vi "Initialize Multicolumn Listbox.vi"(8 "error in":errorcluster, 11 "MulticolumnListbox":refnum<vi>) -> (0 "error out":errorcluster)   [LabVIEW 2018, in "NI_TDMS File Viewer.lvlib"]
uses:
  NI_TDMS File Viewer.lvlib
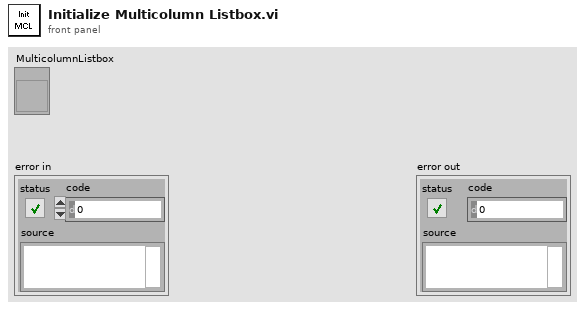
[diagram p1: front panel]
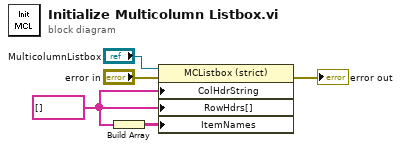
[diagram p0: block diagram]
diagram:
  w3 = string[] [] ("Column Header Strings[]")
  n1 = Build Array(w3) -> (w2:string[][])
  n2 = property on="Property Node" class="MCListbox (strict)"(reference="MulticolumnListbox", error in="error in", "ColHdrString"=w3, "RowHdrs[]"=w3, "ItemNames"=w2) -> (error out=→"error out":errorcluster)  [unwired: 1 out]
